vi "Measurement creator.vi"(0 "Index in":T13={"IV"=[{"Name"="Test", "Comment"="", "Time"=timestamp(0 s since 1904-01-01), "Folder"=path "", "IV properties"={"T"=0.0, "Vstart"=0.0, "Vstop"=0.0, "Vpoints"=0.0, "Settling"=0.01, "I limit"=0.1, "Log mapping"=FALSE, "Averaging"=0.0}, "GUID"=""}], "CV"=[], "LDLTS"=[], "Conv DLTS"=[]} {"IV"."IV properties"."Settling" min=0.0 max=65535.0; "CV"."CV properties"."V range" items=["10mV"=0.01, "100mV"=0.1, "1V"=1.0, "10V"=10.0]; "CV"."CV properties"."I range" items=["100nA"=-7.0, "1µA"=-6.0, "10µA"=-5.0, "100µA"=-4.0, "1mA"=-3.0, "10mA"=-2.0]; "LDLTS"."LDLTS properties"."V range" items=["10mV"=0.01, "100mV"=0.1, "1V"=1.0, "10V"=10.0]; "LDLTS"."LDLTS properties"."I range" items=["100nA"=-7.0, "1µA"=-6.0, "10µA"=-5.0, "100µA"=-4.0, "1mA"=-3.0, "10mA"=-2.0]; "Conv DLTS"."DLTS properties"."V range" items=["10mV"=0.01, "100mV"=0.1, "1V"=1.0, "10V"=10.0]; "Conv DLTS"."DLTS properties"."I range" items=["10mV"=0.01, "100mV"=0.1, "1V"=1.0, "10V"=10.0]}, 5 "Workspace":path, 7 "Settings":T1={"MFIA"={"Address"="", "Use compensation"=TRUE, "Shut down gracefully"=FALSE}, "Temp ctrl"={"Gain (P)"=0.0, "Reset (I)"=0.0, "Rate (D)"=0, "Stabilization rate"=0.0, "Stabilization delta"=0.0, "Type"=enum."Lake Shore 325", "Custom temp ctrl"={"VISA resource name"=""}, "Lakeshore 325"={"VISA name"="", "Loop"=0, "Heater Range"=1, "Heater Resistance"=0, "Sample sensor"=0, "Fast sensor"=0, "Slow sensor"=0}}, "Source-meter"={"Type"=enum."Custom", "Custom source-meter"={"VISA resource name"=""}, "Keithley 2600"={"VISA name"=""}}, "Other"={"Enable OriginLab"=FALSE, "Reader mode"=FALSE}, "Defaults"={"IV properties"={"T"=0.0, "Vstart"=-0.5, "Vstop"=0.5, "Vpoints"=10.0, "Settling"=0.01, "I limit"=0.1, "Log mapping"=FALSE, "Averaging"=0.0}, "CV properties"={"T"=0.0, "Vstart"=-0.5, "Vstop"=0.5, "Vpoints"=10.0, "Precision"=enum."Normal", "Test signal"=0.01, "Auto I range"=FALSE, "Test frequency"=100000.0, "I range"=-2.0, "V range"=10.0, "Log mapping"=FALSE, "Rel perm"=0.0, "Area"=0.0}, "DLTS properties"={"Tstart"=0.0, "Instant start"=FALSE, "Tstop"=0.0, "T rate"=0.0, "Test signal"=0.0, "Test frequency"=0.0, "Bandwidth"=0.0, "Averaging"=0.0, "Vbias"=0.0, "Vpulse"=0.0, "pulse length"=0.0, "Pulse 2"=FALSE, "Vpulse 2"=0.0, "pulse length 2"=0.0, "I range"=-2.0, "V range"=10.0, "Emission rate"=[], "Sampling rate"=0.0, "Acq. delay"=0.0}, "LDLTS properties"={"T"=0.0, "Test signal"=0.0, "Test frequency"=0.0, "Bandwidth"=0.0, "Averaging"=0.0, "Vbias"=0.0, "Vpulse"=0.0, "pulse length"=0.0, "Pulse 2"=FALSE, "Vpulse 2"=0.0, "pulse length 2"=0.0, "I range"=-2.0, "V range"=10.0, "Sampling rate"=0.0, "Acq. delay"=0.0, "Sampling time"=0.0}}} {"Defaults"."LDLTS properties"."V range" items=["10mV"=0.01, "100mV"=0.1, "1V"=1.0, "10V"=10.0]; "Defaults"."LDLTS properties"."I range" items=["100nA"=-7.0, "1µA"=-6.0, "10µA"=-5.0, "100µA"=-4.0, "1mA"=-3.0, "10mA"=-2.0]; "Defaults"."DLTS properties"."V range" items=["10mV"=0.01, "100mV"=0.1, "1V"=1.0, "10V"=10.0]; "Defaults"."DLTS properties"."I range" items=["10mV"=0.01, "100mV"=0.1, "1V"=1.0, "10V"=10.0]; "Defaults"."CV properties"."V range" items=["10mV"=0.01, "100mV"=0.1, "1V"=1.0, "10V"=10.0]; "Defaults"."CV properties"."I range" items=["100nA"=-7.0, "1µA"=-6.0, "10µA"=-5.0, "100µA"=-4.0, "1mA"=-3.0, "10mA"=-2.0]; "Defaults"."IV properties"."Settling" min=0.0 max=65535.0; "Temp ctrl"."Lakeshore 325"."Slow sensor" items=["A", "B"]; "Temp ctrl"."Lakeshore 325"."Fast sensor" items=["A", "B"]; "Temp ctrl"."Lakeshore 325"."Sample sensor" items=["A", "B"]; "Temp ctrl"."Lakeshore 325"."Heater Resistance" items=["25 Ohm"=1, "50 Ohm"=2]; "Temp ctrl"."Lakeshore 325"."Heater Range" items=["Off", "Low (loop 1) or On (loop 2)", "High (loop 1)"]; "Temp ctrl"."Lakeshore 325"."Loop" items=["Loop 1"=1, "Loop 2"=2]}, 11 "error in (no error)":errorcluster) -> (4 "Index out":T13={"IV"=[{"Name"="Test", "Comment"="", "Time"=timestamp(0 s since 1904-01-01), "Folder"=path "", "IV properties"={"T"=0.0, "Vstart"=0.0, "Vstop"=0.0, "Vpoints"=0.0, "Settling"=0.01, "I limit"=0.1, "Log mapping"=FALSE, "Averaging"=0.0}, "GUID"=""}], "CV"=[], "LDLTS"=[], "Conv DLTS"=[]} {"IV"."IV properties"."Settling" min=0.0 max=65535.0; "CV"."CV properties"."V range" items=["10mV"=0.01, "100mV"=0.1, "1V"=1.0, "10V"=10.0]; "CV"."CV properties"."I range" items=["100nA"=-7.0, "1µA"=-6.0, "10µA"=-5.0, "100µA"=-4.0, "1mA"=-3.0, "10mA"=-2.0]; "LDLTS"."LDLTS properties"."V range" items=["10mV"=0.01, "100mV"=0.1, "1V"=1.0, "10V"=10.0]; "LDLTS"."LDLTS properties"."I range" items=["100nA"=-7.0, "1µA"=-6.0, "10µA"=-5.0, "100µA"=-4.0, "1mA"=-3.0, "10mA"=-2.0]; "Conv DLTS"."DLTS properties"."V range" items=["10mV"=0.01, "100mV"=0.1, "1V"=1.0, "10V"=10.0]; "Conv DLTS"."DLTS properties"."I range" items=["10mV"=0.01, "100mV"=0.1, "1V"=1.0, "10V"=10.0]}, 6 "ID":i32, 8 "Type":enum16{"I-V", "C-V", "cDLTS", "LDLTS"}(ring), 10 "Canceled":bool, 15 "error out":errorcluster)   [LabVIEW 2019]
doc: "Handles creation of a new measurement, displays a GUI window"
uses:
  Type defs/Session internal index Type Def.ctl
  Type defs/IV measurement Type Def.ctl
  Type defs/IV properties Type Def.ctl
  Type defs/CV measurement Type Def.ctl
  Type defs/CV properties Type Def.ctl
  Type defs/LDLTS measurement Type Def.ctl
  Type defs/LDLTS properties Type Def.ctl
  Type defs/cDLTS measurement Type Def.ctl
  Type defs/DLTS properties Type Def.ctl
  Type defs/Settings Type Def.ctl
  Type defs/Imps Type Def.ctl
  Type defs/Temp ctrl Type Def.ctl
  Custom devices/Custom temp ctrl settings.ctl
  Type defs/Source-meter Type Def.ctl
  Custom devices/Custom source-meter settings.ctl
  Type defs/Other settings Type Def.ctl
  <vilib>/Utility/miscctls.llb/LVPointTypeDef.ctl
panel:
  in  "Type ctrl":T12(ring)=enum."C-V" caption="Measurement type"
  in  "Cancel":bool
  in  "Apply":bool
  in  "Comment":string
  in  "Measurment name":string
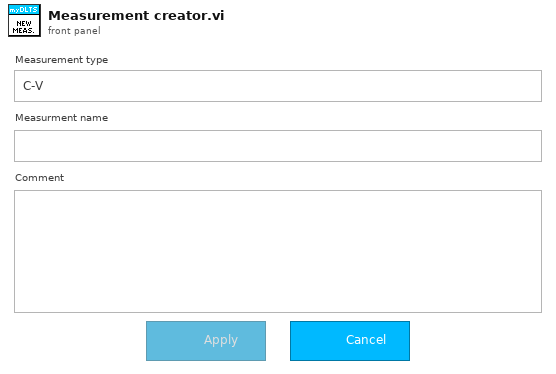
[diagram p1: front panel]
types:
  T1 = typedef "Settings Type Def.ctl" = cluster{"MFIA":T2, "Temp ctrl":T3, "Source-meter":T5, "Other":T7, "Defaults":cluster{"IV properties":T8, "CV properties":T9, "DLTS properties":T10, "LDLTS properties":T11}}
  T2 = typedef "Imps Type Def.ctl" = cluster{"Address":string, "Use compensation":bool, "Shut down gracefully":bool}
  T3 = typedef "Temp ctrl Type Def.ctl" = cluster{"Gain (P)":dbl, "Reset (I)":dbl, "Rate (D)":u16, "Stabilization rate":dbl, "Stabilization delta":dbl, "Type":enum16{"Custom", "Lake Shore 325"}, "Custom temp ctrl":T4, "Lakeshore 325":cluster{"VISA name":refnum<visa-resource-name>, "Loop":u16, "Heater Range":u16, "Heater Resistance":u16, "Sample sensor":u16, "Fast sensor":u16, "Slow sensor":u16}}
  T4 = typedef "Custom temp ctrl settings.ctl" = cluster{"VISA resource name":refnum<visa-resource-name>}
  T5 = typedef "Source-meter Type Def.ctl" = cluster{"Type":enum16{"Custom", "Keithley 2600"}, "Custom source-meter":T6, "Keithley 2600":cluster{"VISA name":refnum<visa-resource-name>}}
  T6 = typedef "Custom source-meter settings.ctl" = cluster{"VISA resource name":refnum<visa-resource-name>}
  T7 = typedef "Other settings Type Def.ctl" = cluster{"Enable OriginLab":bool, "Reader mode":bool}
  T8 = typedef "IV properties Type Def.ctl" = cluster{"T":dbl[unit], "Vstart":dbl[unit], "Vstop":dbl[unit], "Vpoints":dbl, "Settling":dbl[unit], "I limit":dbl[unit], "Log mapping":bool, "Averaging":dbl}
  T9 = typedef "CV properties Type Def.ctl" = cluster{"T":dbl[unit], "Vstart":dbl[unit], "Vstop":dbl[unit], "Vpoints":dbl, "Precision":enum16{"Low (Fast)", "Normal", "High (Slow)"}, "Test signal":dbl[unit], "Auto I range":bool, "Test frequency":dbl[unit], "I range":dbl, "V range":dbl[unit], "Log mapping":bool, "Rel perm":dbl, "Area":dbl[unit]}
  T10 = typedef "DLTS properties Type Def.ctl" = cluster{"Tstart":dbl[unit], "Instant start":bool, "Tstop":dbl[unit], "T rate":dbl[unit], "Test signal":dbl[unit], "Test frequency":dbl[unit], "Bandwidth":dbl[unit], "Averaging":dbl, "Vbias":dbl[unit], "Vpulse":dbl[unit], "pulse length":dbl[unit], "Pulse 2":bool, "Vpulse 2":dbl[unit], "pulse length 2":dbl[unit], "I range":dbl, "V range":dbl[unit], "Emission rate":dbl[unit][], "Sampling rate":dbl[unit], "Acq. delay":dbl[unit]}
  T11 = typedef "LDLTS properties Type Def.ctl" = cluster{"T":dbl[unit], "Test signal":dbl[unit], "Test frequency":dbl[unit], "Bandwidth":dbl[unit], "Averaging":dbl, "Vbias":dbl[unit], "Vpulse":dbl[unit], "pulse length":dbl[unit], "Pulse 2":bool, "Vpulse 2":dbl[unit], "pulse length 2":dbl[unit], "I range":dbl, "V range":dbl[unit], "Sampling rate":dbl[unit], "Acq. delay":dbl[unit], "Sampling time":dbl[unit]}
  T12 = enum16{"I-V", "C-V", "Conventional DLTS", "Laplace DLTS"}
  T13 = typedef "Session internal index Type Def.ctl" = cluster{"IV":T14[], "CV":T15[], "LDLTS":T16[], "Conv DLTS":T17[]}
  T14 = typedef "IV measurement Type Def.ctl" = cluster{"Name":string, "Comment":string, "Time":timestamp, "Folder":path, "IV properties":T8, "GUID":string}
  T15 = typedef "CV measurement Type Def.ctl" = cluster{"Name":string, "Comment":string, "Time":timestamp, "Folder":path, "CV properties":T9, "GUID":string}
  T16 = typedef "LDLTS measurement Type Def.ctl" = cluster{"Name":string, "Comment":string, "Time":timestamp, "Folder":path, "LDLTS properties":T11, "GUID":string}
  T17 = typedef "cDLTS measurement Type Def.ctl" = cluster{"Name":string, "Comment":string, "Time":timestamp, "Folder":path, "DLTS properties":T10, "GUID":string}
  T18 = enum8{"Enabled", "Disabled", "Disabled and Grayed Out"}
  T19 = typedef "LVPointTypeDef.ctl" = cluster{"Horizontal":i16, "Vertical":i16}
  T20 = cluster{"IV properties":T8, "CV properties":T9, "DLTS properties":T10, "LDLTS properties":T11}
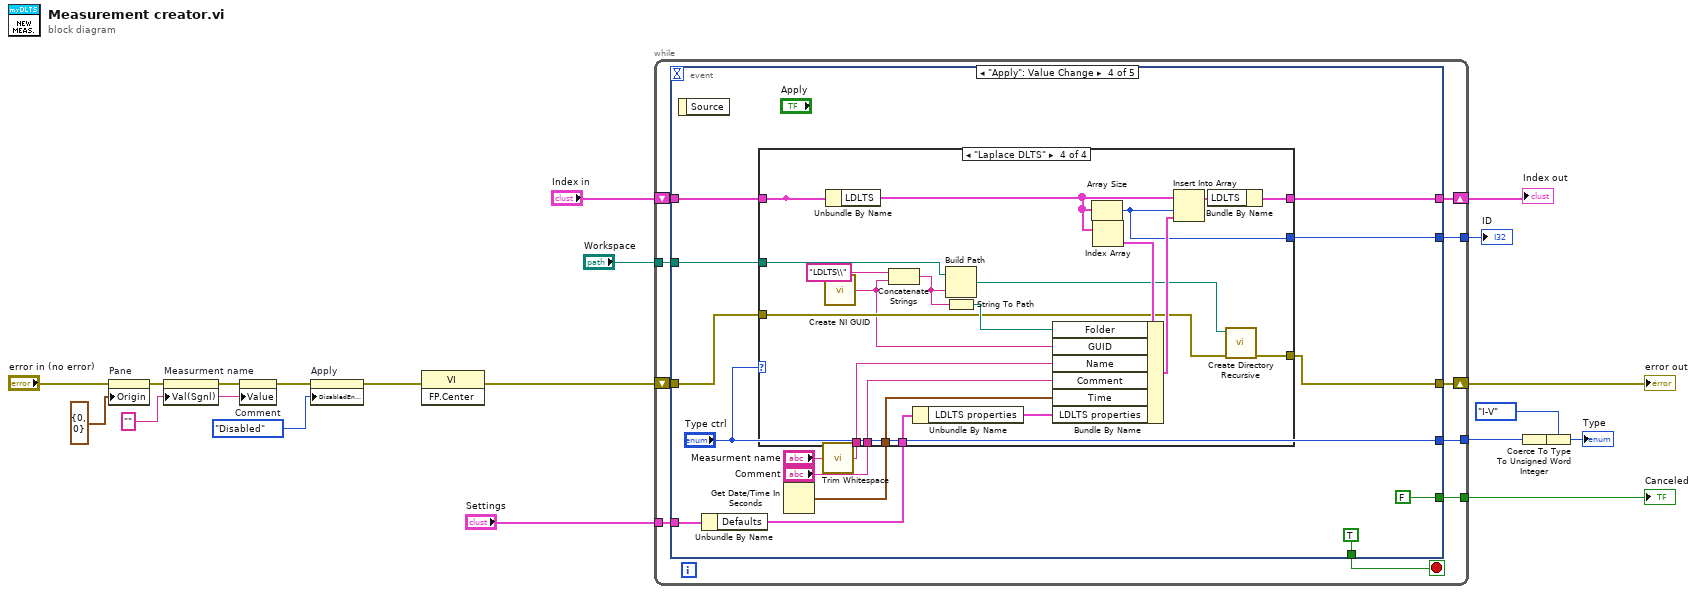
[diagram p0: block diagram]
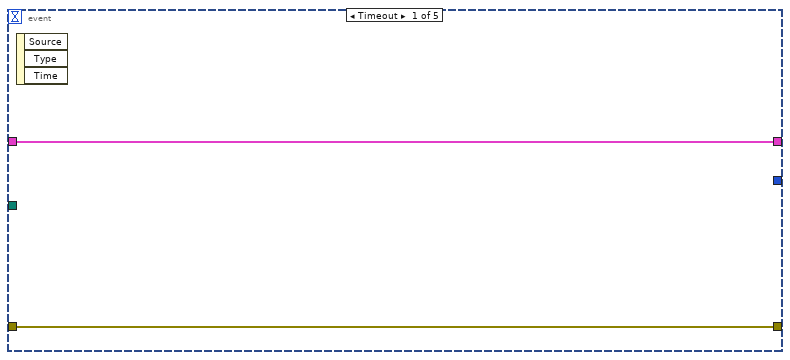
[diagram p2: hidden frame]
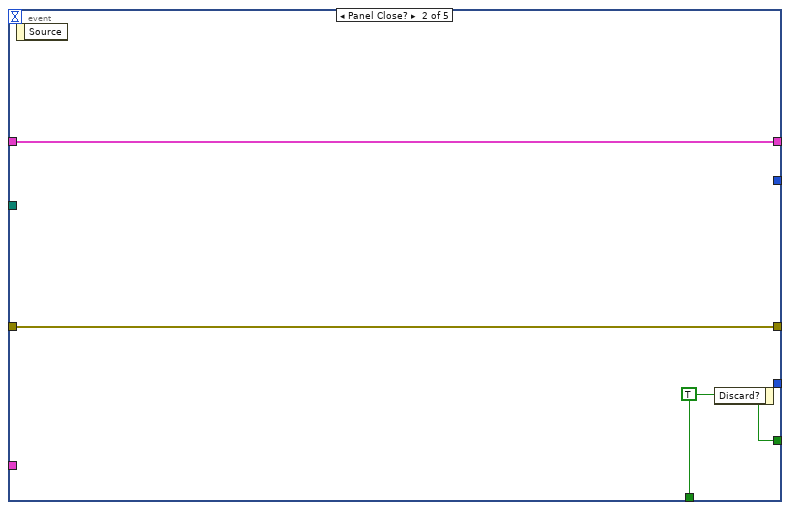
[diagram p3: hidden frame]
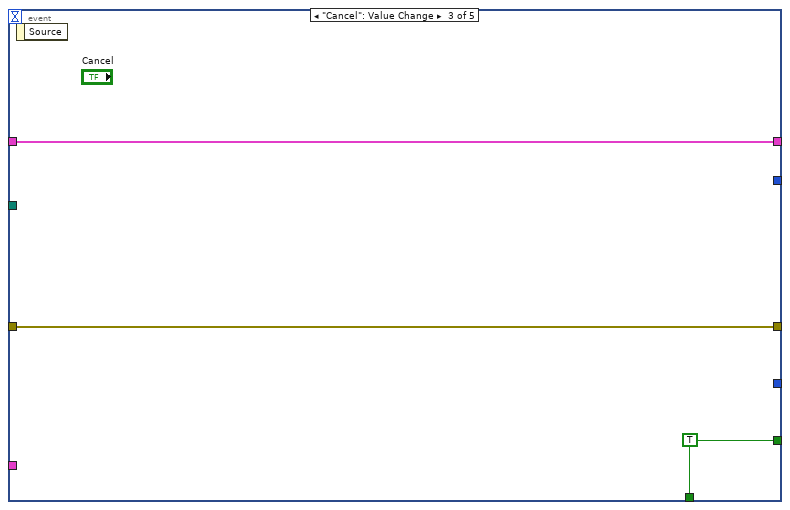
[diagram p4: hidden frame]
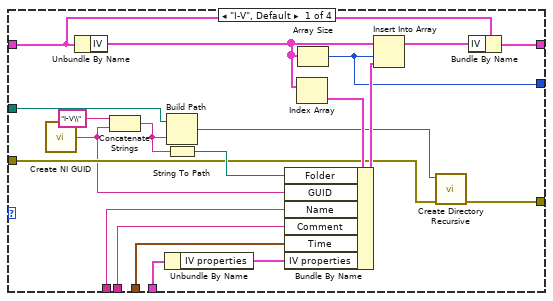
[diagram p5: hidden frame]
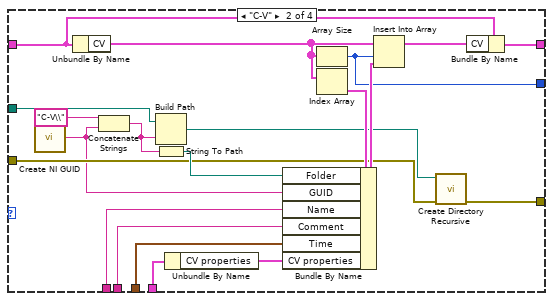
[diagram p6: hidden frame]
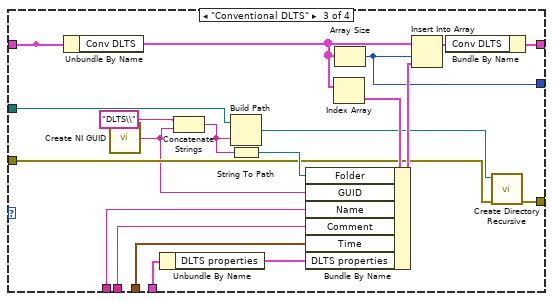
[diagram p7: hidden frame]
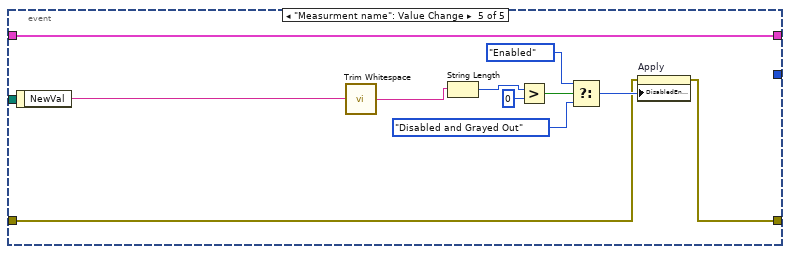
[diagram p8: hidden frame]
diagram:
  w14 = "" ("Value (Signaling)")
  n1 = property on="Pane" class="Pane"(error in="error in (no error)", "Origin"=T19 {"Horizontal"=0, "Vertical"=0}) -> (error out=w19:errorcluster)  [unwired: 1 in, 1 out]
  n2 = property on="Measurment name" class="Str"(error in=w19, "Val(Sgnl)"=w14) -> (error out=w15:errorcluster)  [unwired: 1 in, 1 out]
  n3 = property on="Comment" class="Str"(error in=w15, "Value"=w14) -> (error out=w12:errorcluster)  [unwired: 1 in, 1 out]
  n4 = property on="Apply" class="Bool"(error in=w12, "DisabledEnum"=T18."Disabled" ("Disabled")) -> (error out=w7:errorcluster)  [unwired: 1 in, 1 out]
  n5 = invoke class="VI" method="FP.Center"(error in=w7) -> (error out=w6:errorcluster)  [unwired: 2 in, 2 out]
  n6 = while {
    tunnel: [w29] -> w20
    shift-right: [w27] -> w17
    shift-left: w6 -> [w28]
    tunnel: "Workspace" -> [w25]
    tunnel: [w23] -> w8
    shift-right: [w24] -> w9
    shift-left: "Index in" -> [w26]
    tunnel: [w22] -> w5
    tunnel: "Settings" -> [w21]
    stop <- w30 stop-if-true
    n7 = event shown="[3] \"Apply\": Value Change" {
      selector: _ -> [_ _ _ _ _]
      dyn-events: _ -> [_ _ _ _ _]
      timeout: _ -> [_ _ _ _ _]
      tunnel: [_ w35 w38 TRUE ("Discard?") _] -> w30
      tunnel: [_ w35 w38 FALSE ("Discard?") _] -> w29
      tunnel: w28 -> [w32 w34 w37 w42 w139]
      tunnel: [w32 w34 w37 w44 w140] -> w27
      tunnel: w26 -> [w31 w33 w36 w50 w134]
      tunnel: w25 -> [_ _ _ w46 _]
      tunnel: [w31 w33 w36 w45 w134] -> w24
      tunnel: [_ _ _ w43 _] -> w23
      tunnel: [_ _ _ "Type ctrl" _] -> w22
      tunnel: w21 -> [_ _ _ w40 _]
      event Timeout {
        n8 = event-data() -> ()  [unwired: 1 in, 3 out]
      }
      event Panel Close? {
        w35 = TRUE ("Discard?")
        n9 = event-data() -> ()  [unwired: 1 in, 1 out]
        n10 = event-data("Discard?"=w35) -> ()  [unwired: 1 in, 1 out]
      }
      event "Cancel": Value Change {
        w38 = TRUE ("Discard?")
        n11 = event-data() -> ()  [unwired: 1 in, 1 out]
      }
      event "Apply": Value Change {
        n12 = event-data() -> ()  [unwired: 1 in, 1 out]
        n13 = Unbundle By Name(w40) -> ("Defaults"=w39:T20)
        n14 = Get Date/Time In Seconds() -> (seconds since 1Jan1904=w47:timestamp)
        n15 = call <vilib>:"Trim Whitespace.vi"("string"="Measurment name") -> ("trimmed string"=w49:string)  [unwired: 1 in]
        n16 = case shown="\"Laplace DLTS\"" "Type ctrl" {
          tunnel: w50 -> [w66 w86 w106 w126]
          tunnel: w49 -> [w73 w93 w113 w133]
          tunnel: "Comment" -> [w72 w92 w112 w132]
          tunnel: w47 -> [w70 w90 w110 w130]
          tunnel: w46 -> [w56 w76 w98 w121]
          tunnel: [w65 w85 w105 w125] -> w45
          tunnel: [w67 w87 w107 w127] -> w44
          tunnel: [w63 w83 w103 w123] -> w43
          tunnel: w42 -> [w55 w77 w95 w115]
          tunnel: w39 -> [w62 w82 w102 w120]
          frame "I-V", Default {
            n17 = call "Create NI GUID.vi"() -> ("NI GUID"=w54:string)
            n18 = Unbundle By Name(w66) -> ("IV"=w68:T14[])
            n19 = Concatenate Strings("I-V\\" ("string"), w54) -> (w60:string)
            n20 = Unbundle By Name(w62) -> ("IV properties"=w61:T8)
            n21 = Build Path(base path=w56, name or relative path=w60) -> (appended path=w57:path)
            n22 = String To Path(string=w60) -> (path=w58:path)
            n23 = Index Array(array=w68) -> (element=w71:T14)  [unwired: 1 in]
            n24 = Bundle By Name(cluster=w71, "Folder"=w58, "GUID"=w54, "Name"=w73, "Comment"=w72, "Time"=w70, "IV properties"=w61) -> (w69:T14)
            n25 = Array Size(array=w68) -> (size(s)=w63:i32)
            n26 = Insert Into Array(array=w68, index=w63, new element=w69) -> (w64:T14[])
            n27 = call <vilib>:"Create Directory Recursive.vi"("error in (no error)"=w55, "directory"=w57) -> ("error out"=w67:errorcluster)  [unwired: 3 in, 2 out]
            n28 = Bundle By Name(cluster=w66, "IV"=w64) -> (w65:T13)
          }
          frame "C-V" {
            n29 = call "Create NI GUID.vi"() -> ("NI GUID"=w74:string)
            n30 = Unbundle By Name(w86) -> ("CV"=w88:T15[])
            n31 = Concatenate Strings("C-V\\" ("string"), w74) -> (w80:string)
            n32 = Build Path(base path=w76, name or relative path=w80) -> (appended path=w75:path)
            n33 = String To Path(string=w80) -> (path=w78:path)
            n34 = Unbundle By Name(w82) -> ("CV properties"=w81:T9)
            n35 = Array Size(array=w88) -> (size(s)=w83:i32)
            n36 = Index Array(array=w88) -> (element=w91:T15)  [unwired: 1 in]
            n37 = Bundle By Name(cluster=w91, "Folder"=w78, "GUID"=w74, "Name"=w93, "Comment"=w92, "Time"=w90, "CV properties"=w81) -> (w89:T15)
            n38 = Insert Into Array(array=w88, index=w83, new element=w89) -> (w84:T15[])
            n39 = call <vilib>:"Create Directory Recursive.vi"("error in (no error)"=w77, "directory"=w75) -> ("error out"=w87:errorcluster)  [unwired: 3 in, 2 out]
            n40 = Bundle By Name(cluster=w86, "CV"=w84) -> (w85:T13)
          }
          frame "Conventional DLTS" {
            n41 = Unbundle By Name(w106) -> ("Conv DLTS"=w108:T17[])
            n42 = call "Create NI GUID.vi"() -> ("NI GUID"=w94:string)
            n43 = Unbundle By Name(w102) -> ("DLTS properties"=w101:T10)
            n44 = Concatenate Strings("DLTS\\" ("string"), w94) -> (w100:string)
            n45 = Build Path(base path=w98, name or relative path=w100) -> (appended path=w97:path)
            n46 = String To Path(string=w100) -> (path=w96:path)
            n47 = Index Array(array=w108) -> (element=w111:T17)  [unwired: 1 in]
            n48 = Bundle By Name(cluster=w111, "Folder"=w96, "GUID"=w94, "Name"=w113, "Comment"=w112, "Time"=w110, "DLTS properties"=w101) -> (w109:T17)
            n49 = Array Size(array=w108) -> (size(s)=w103:i32)
            n50 = Insert Into Array(array=w108, index=w103, new element=w109) -> (w104:T17[])
            n51 = Bundle By Name(cluster=w106, "Conv DLTS"=w104) -> (w105:T13)
            n52 = call <vilib>:"Create Directory Recursive.vi"("error in (no error)"=w95, "directory"=w97) -> ("error out"=w107:errorcluster)  [unwired: 3 in, 2 out]
          }
          frame "Laplace DLTS" {
            n53 = call "Create NI GUID.vi"() -> ("NI GUID"=w114:string)
            n54 = Unbundle By Name(w126) -> ("LDLTS"=w128:T16[])
            n55 = Concatenate Strings("LDLTS\\" ("string"), w114) -> (w117:string)
            n56 = Unbundle By Name(w120) -> ("LDLTS properties"=w119:T11)
            n57 = Build Path(base path=w121, name or relative path=w117) -> (appended path=w118:path)
            n58 = String To Path(string=w117) -> (path=w122:path)
            n59 = Array Size(array=w128) -> (size(s)=w123:i32)
            n60 = Index Array(array=w128) -> (element=w131:T16)  [unwired: 1 in]
            n61 = Bundle By Name(cluster=w131, "Folder"=w122, "GUID"=w114, "Name"=w133, "Comment"=w132, "Time"=w130, "LDLTS properties"=w119) -> (w129:T16)
            n62 = Insert Into Array(array=w128, index=w123, new element=w129) -> (w124:T16[])
            n63 = Bundle By Name(cluster=w126, "LDLTS"=w124) -> (w125:T13)
            n64 = call <vilib>:"Create Directory Recursive.vi"("error in (no error)"=w115, "directory"=w118) -> ("error out"=w127:errorcluster)  [unwired: 3 in, 2 out]
          }
        }
      }
      event "Measurment name": Value Change {
        n65 = event-data() -> ("NewVal"=w142:string)  [unwired: 1 in]
        n66 = call <vilib>:"Trim Whitespace.vi"("string"=w142) -> ("trimmed string"=w138:string)  [unwired: 1 in]
        n67 = String Length(string=w138) -> (length=w136:i32)
        n68 = Greater?(x=w136, y=0) -> (0:w135:bool)
        n69 = Select(t=T18."Enabled" ("Disabled"), s=w135, f=T18."Disabled and Grayed Out") -> (s? t:f=w141:T18)
        n70 = property on="Apply" class="Bool"(error in=w139, "DisabledEnum"=w141) -> (error out=w140:errorcluster)  [unwired: 1 in, 1 out]
      }
    }
  }
  "Canceled" <- w20
  "error out" <- w17
  "Index out" <- w9
  "ID" <- w8
  n71 = To Unsigned Word Integer(number=w5) -> (unsigned 16bit integer=w4:u16)
  n72 = Coerce To Type(0:w4, 1:enum16{"I-V", "C-V", "cDLTS", "LDLTS"}."I-V" ("Type")) -> (2:→"Type":enum16{"I-V", "C-V", "cDLTS", "LDLTS"})
